vi "UDP Data Link - Configuration Utilities - Evaluate Tx Imported Channels.vi"(8 "error in (no error)":errorcluster, 9 "Section Info":T1, 10 "Channel Info Array":T2[](array[typedef]) {"Data Type" items=["U8", "U16", "U32", "U64", "I8", "I16", "I32", "I64", "SGL", "DBL", "EXT"]}, 11 "Node Ptr in":u64 format="%.0x") -> (0 "error out":errorcluster, 2 "Invalid Channels":string[](array[string]), 3 "Node Ptr out":u64 format="%.0x")   [LabVIEW 2015, in "UDP-Custom-Device System Explorer.lvlib"]
uses:
  UDP-Custom-Device System Explorer.lvlib
  Types/UDP Data Link - TypeDefs - XML Channel.ctl
  Types/UDP Data Link - TypeDefs - Section Info.ctl
  <vilib>/NI Veristand/Custom Device API/Custom Device Item Ref.ctl
  <vilib>/NI Veristand/Custom Device Tools/Custom Device Utility Library/NI VeriStand - Search for Item by GUID.vi
  <vilib>/NI Veristand/Custom Device API/Get Item Property (String Array).vi
  <vilib>/NI Veristand/Custom Device API/Set Item Property (String Array).vi
  <vilib>/NI VeriStand/Custom Device Tools/Custom Device Utility Library/Custom Device Utility Library.lvlib
  <vilib>/NI VeriStand/Custom Device API/Custom Device API.lvlib
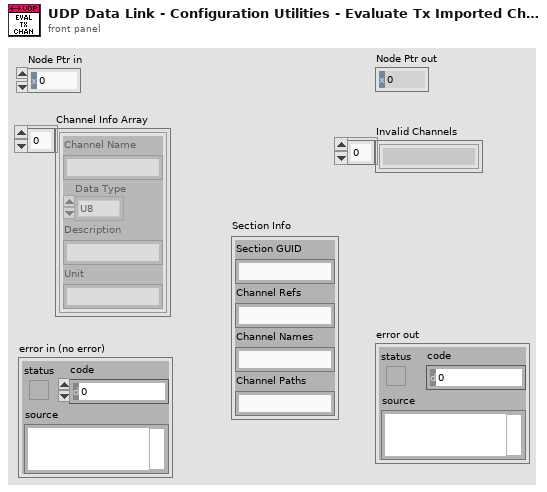
[diagram p1: front panel]
types:
  T1 = typedef "UDP-Custom-Device System Explorer.lvlib/UDP Data Link - TypeDefs - Section Info.ctl" = cluster{"Section GUID":string, "Channel Refs":string, "Channel Names":string, "Channel Paths":string}
  T2 = typedef "UDP-Custom-Device System Explorer.lvlib/UDP Data Link - TypeDefs - XML Channel.ctl" = cluster{"Channel Name":string, "Data Type":u16, "Description":string, "Unit":string}
  T3 = typedef "Custom Device API.lvlib/Custom Device Item Ref.ctl" = u64
  T4 = typedef "Custom Device API.lvlib/Custom Device Item Info.ctl" = cluster{"Name":string, "Is Channel":bool, "GUID":string, "Is Waveform":bool}
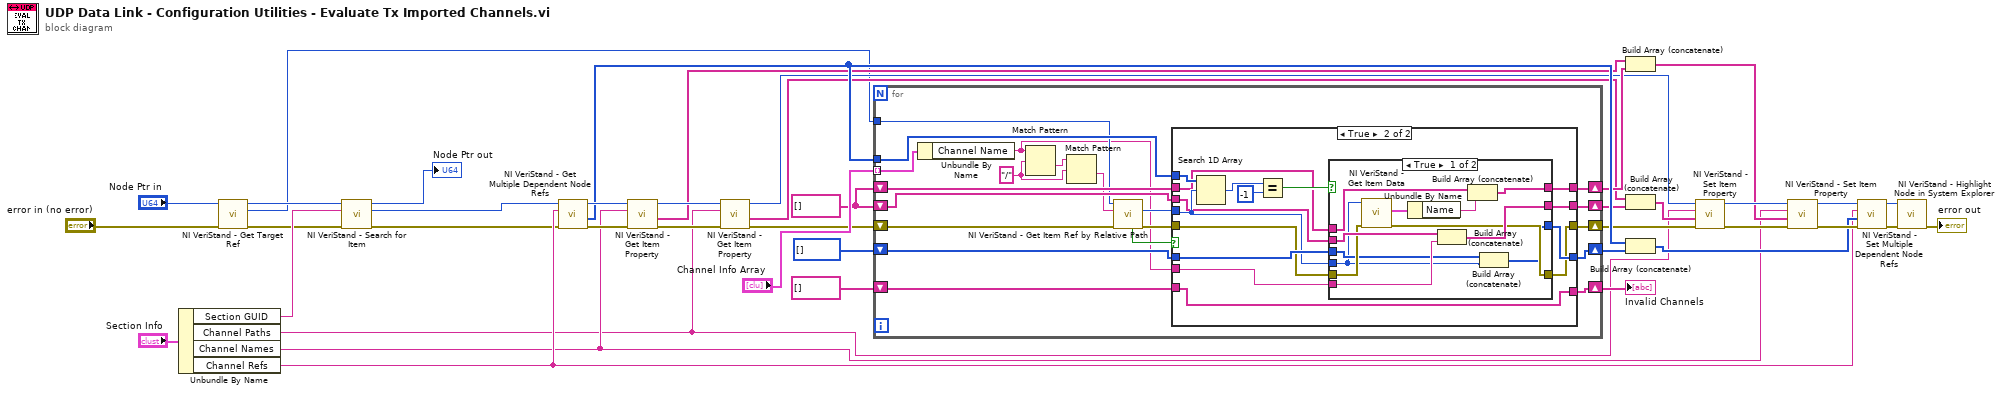
[diagram p0: block diagram]
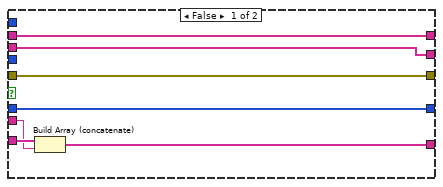
[diagram p2: hidden frame]
diagram:
  w31 = string[] []
  n1 = Unbundle By Name("Section Info") -> ("Section GUID"=w11:string, "Channel Paths"=w8:string, "Channel Names"=w9:string, "Channel Refs"=w10:string)
  n2 = call <vilib>:"NI VeriStand - Get Target Ref.vi"("error in"="error in (no error)", "Item Ref in"="Node Ptr in") -> ("error out"=w6:errorcluster, "Target Ref"=w3:T3, "Item Ref out"=w4:T3)  [unwired: 6 in, 1 out]
  n3 = call-poly <vilib>:"NI VeriStand - Search for Item.vi"("error in"=w6, "Item GUID"=w11, "Section Ref in"=w4) -> ("error out"=w2:errorcluster, "Item Ref"=w1:T3, "Section Ref out"=→"Node Ptr out":T3)  [unwired: 5 in, 1 out]
  n4 = call <vilib>:"NI VeriStand - Get Multiple Dependent Node Refs.vi"("error in (no error)"=w2, "Base Property Name"=w10, "Item Ref in"=w1) -> ("error out"=w37:errorcluster, "Dependent Node Refs"=w30:T3[], "Item Ref out"=w36:T3)  [unwired: 6 in]
  n5 = call-poly <vilib>:"NI VeriStand - Get Item Property.vi"("error in (no error)"=w37, "Property Name"=w9, "Item Ref in"=w36) -> ("error out"=w35:errorcluster, "Value"=w28:string[], "Item Ref out"=w34:T3)  [unwired: 5 in, 1 out]
  n6 = call-poly <vilib>:"NI VeriStand - Get Item Property.vi"("error in (no error)"=w35, "Property Name"=w8, "Item Ref in"=w34) -> ("error out"=w33:errorcluster, "Value"=w26:string[], "Item Ref out"=w23:T3)  [unwired: 5 in, 1 out]
  n7 = for {
    tunnel: "Channel Info Array" -> [w61] mode=indexing
    shift-right: [w60] -> w24
    shift-left: w33 -> [w50]
    shift-right: [w58] -> w39
    shift-left: string[] [] -> [w59]
    tunnel: w30 -> [w57]
    shift-right: [w55] -> w29
    shift-left: T3[] [] -> [w56]
    shift-right: [w53] -> w27
    shift-left: w31 -> [w54]
    shift-right: [w51] -> w25
    shift-left: w31 -> [w52]
    tunnel: w3 -> [w48]
    w43 = "/" ("regular expression")
    n8 = Unbundle By Name(w61) -> ("Channel Name"=w45:string)
    n9 = Match Pattern(string=w45, regular expression=w43) -> (after substring=w44:string)  [unwired: 1 in, 3 out]
    n10 = Match Pattern(string=w44, regular expression=w43) -> (after substring=w42:string)  [unwired: 1 in, 3 out]
    n11 = call <vilib>:"NI VeriStand - Get Item Ref by Relative Path.vi"("error in"=w50, "Relative Item Path"=w42, "Section Ref in"=w48) -> ("error out"=w49:errorcluster, "Item Ref"=w47:T3, "Found"=w46:bool)  [unwired: 5 in, 1 out]
    n12 = case shown="True" w46 {
      tunnel: w49 -> [w65 w75]
      tunnel: [w65 w70] -> w60
      tunnel: w59 -> [w68 w83]
      tunnel: w45 -> [w67 w69]
      tunnel: [w66 w83] -> w58
      tunnel: w57 -> [_ w82]
      tunnel: w47 -> [_ w77]
      tunnel: w56 -> [w64 w78]
      tunnel: [w64 w76] -> w55
      tunnel: w54 -> [w63 w74]
      tunnel: [w63 w73] -> w53
      tunnel: w52 -> [w62 w72]
      tunnel: [w62 w71] -> w51
      frame False {
        n13 = Build Array (concatenate)(w68, w67) -> (w66:string[])
      }
      frame True {
        n14 = Search 1D Array(1D array=w82, element=w77) -> (index of element=w81:i32)  [unwired: 1 in]
        n15 = Equal?(x=w81, y=-1) -> (x = y?=w79:bool)
        n16 = case shown="True" w79 {
          tunnel: w78 -> [w86 w98]
          tunnel: w77 -> [w85 _]
          tunnel: [w84 w98] -> w76
          tunnel: w75 -> [w92 w99]
          tunnel: w74 -> [w88 w97]
          tunnel: [w87 w97] -> w73
          tunnel: w72 -> [w93 w96]
          tunnel: [w94 w96] -> w71
          tunnel: [w91 w99] -> w70
          tunnel: w69 -> [w95 _]
          frame True {
            n17 = call <vilib>:"NI VeriStand - Get Item Data.vi"("error in (no error)"=w92, "Item Ref in"=w85) -> ("error out"=w91:errorcluster, "Item Info"=w90:T4)  [unwired: 6 in, 2 out]
            n18 = Unbundle By Name(w90) -> ("Name"=w89:string)
            n19 = Build Array (concatenate)(w93, w95) -> (w94:string[])
            n20 = Build Array (concatenate)(w88, w89) -> (w87:string[])
            n21 = Build Array (concatenate)(w86, w85) -> (w84:T3[])
          }
          frame False {
          }
        }
      }
    }
  }
  "Invalid Channels" <- w39
  n22 = Build Array (concatenate)(w28, w27) -> (w20:string[])
  n23 = Build Array (concatenate)(w26, w25) -> (w22:string[])
  n24 = Build Array (concatenate)(w30, w29) -> (w16:T3[])
  n25 = call-poly <vilib>:"NI VeriStand - Set Item Property.vi"("error in (no error)"=w24, "Value"=w22, "Property Name"=w8, "Item Ref in"=w23) -> ("error out"=w19:errorcluster, "Item Ref out"=w21:T3)  [unwired: 5 in, 1 out]
  n26 = call-poly <vilib>:"NI VeriStand - Set Item Property.vi"("error in (no error)"=w19, "Value"=w20, "Property Name"=w9, "Item Ref in"=w21) -> ("error out"=w18:errorcluster, "Item Ref out"=w17:T3)  [unwired: 5 in, 1 out]
  n27 = call <vilib>:"NI VeriStand - Set Multiple Dependent Node Refs.vi"("error in (no error)"=w18, "Dependent Node Refs"=w16, "Base Property Name"=w10, "Item Ref in"=w17) -> ("error out"=w15:errorcluster, "Item Ref out"=w14:T3)  [unwired: 6 in]
  n28 = call <vilib>:"NI VeriStand - Highlight Node in System Explorer.vi"("error in (no error)"=w15, "Item Ref in"=w14) -> ("error out"=→"error out":errorcluster)  [unwired: 8 in, 1 out]
